vi "add_amp_char_to_report.vi"(8 "error in (no error)":errorcluster, 11 "Report in":refnum<class "Report.lvclass">) -> (0 "error out":errorcluster, 3 "Report out":refnum<class "Report.lvclass">)   [LabVIEW 2017, in "Report.lvclass"]
uses:
  Report.lvclass
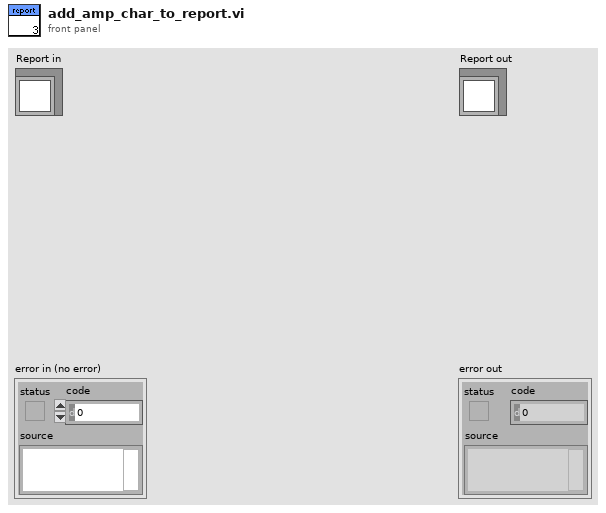
[diagram p1: front panel]
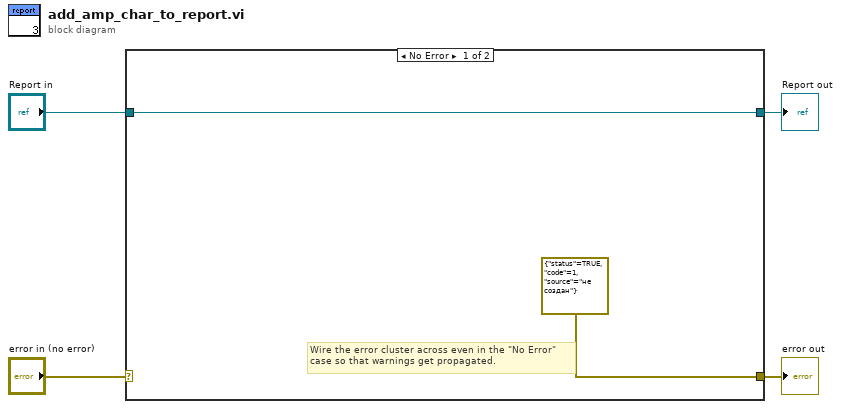
[diagram p0: block diagram]
diagram:
  n1 = case shown="No Error" "error in (no error)" {
    selector: "error in (no error)" -> [_ w8]
    tunnel: [errorcluster {"status"=TRUE, "code"=1, "source"="не создан"} ("error IO") w8] -> w3
    tunnel: [w6 w7] -> w1
    tunnel: "Report in" -> [w6 w7]
    frame No Error {
      # "Wire the error cluster across even in the \"No Error\"\ncase so that warnings get propagated."
    }
    frame Error {
    }
  }
  "error out" <- w3
  "Report out" <- w1
